vi "New Panel Launched.vi"(8 "error in (no error)":errorcluster, 9 "Name":string, 10 "VI Refnum":refnum<vi>, 11 "Chat Window Model in":refnum<class "Chat Window Model.lvclass">) -> (0 "error out":errorcluster, 3 "Chat Window Model out":refnum<class "Chat Window Model.lvclass">)   [LabVIEW 2020, in "Chat Window Model.lvlib" / "Chat Window Model.lvclass"]
uses:
  Chat Window Model.lvclass
  C:/Program Files/National Instruments/LabVIEW 2020/vi.lib/ActorFramework/Actor/Actor.lvclass
  Event-Source-Actor/Data Interface/VI Info Data/VI Info Data.lvclass
  C:/Users/huipeng8/Desktop/SubPanel-Actor-Framework-master/Event-Source-Actor/Source/Template Source/Event Data/Event Data.lvclass
  <vilib>/ActorFramework/Actor/Actor.lvclass/Actor.ctl
  <vilib>/ActorFramework/Message Enqueuer/Message Enqueuer.lvclass/Message Enqueuer.ctl
  SubPanel-Actor-Framework-master/Event-Source-Actor/Source/Template Source/Event Source Messages/Generate Event Msg/Generate Event Msg.lvclass/Generate Event Msg.ctl
  <vilib>/ActorFramework/Message Enqueuer/Init from Existing Queue.vi
  <vilib>/ActorFramework/Message Enqueuer/Enqueue.vi
  SubPanel-Actor-Framework-master/Event-Source-Actor/Source/Template Source/Event Source Messages/Generate Event Msg/Generate Event Msg.lvclass
  C:/Program Files/National Instruments/LabVIEW 2020/vi.lib/ActorFramework/Message/Message.lvclass
  <vilib>/ActorFramework/Message Priority Queue/Priority Enqueue.vi
  <vilib>/ActorFramework/Message Enqueuer/Message Enqueuer.lvclass
  <vilib>/ActorFramework/Actor/Actor.lvclass
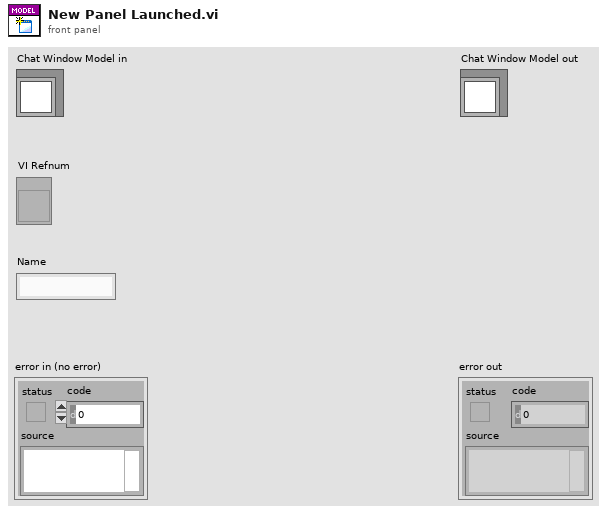
[diagram p1: front panel]
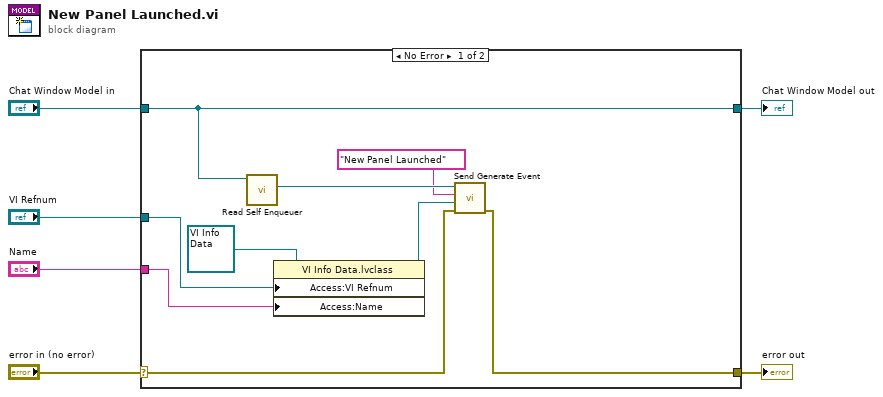
[diagram p0: block diagram]
diagram:
  n1 = case shown="No Error" "error in (no error)" {
    selector: "error in (no error)" -> [w8 w17]
    tunnel: [w7 w17] -> w5
    tunnel: [w15 w16] -> w3
    tunnel: "Chat Window Model in" -> [w15 w16]
    tunnel: "VI Refnum" -> [w10 _]
    tunnel: "Name" -> [w9 _]
    frame No Error {
      n2 = call <vilib>:"Read Self Enqueuer.vi"("Actor"=w15) -> ("Self Enqueuer"=w14:refnum<class "Message Enqueuer.lvclass">)  [unwired: 10 in]
      n3 = property class="VI Info Data.lvclass"(reference=refnum<class "VI Info Data.lvclass"> refnum ("VI Info Data.lvclass"), "Access:VI Refnum"=w10, "Access:Name"=w9) -> (reference out=w11:refnum<class "VI Info Data.lvclass">)  [unwired: 1 in, 1 out]
      n4 = call "Send Generate Event.vi"("error in"=w8, "Event Data"=w11, "Event Name"="New Panel Launched", "Message Enqueuer"=w14) -> ("error out"=w7:errorcluster)  [unwired: 6 in, 1 out]
    }
    frame Error {
    }
  }
  "error out" <- w5
  "Chat Window Model out" <- w3
